vi "VAJ velocity in timing count.vi"(8 "dt":dbl, 9 "time":i32, 11 "Array":cluster{"Numeric":dbl, "Numeric":dbl}[](array[cluster])) -> (0 "t4?":bool, 2 "velocity(cm/s)":dbl, 4 "finish":bool)   [LabVIEW 2019]
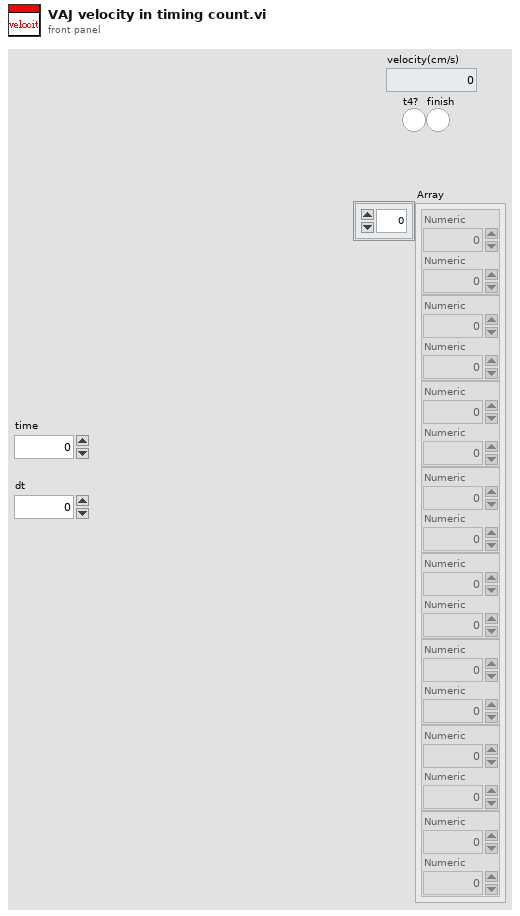
[diagram p1: front panel]
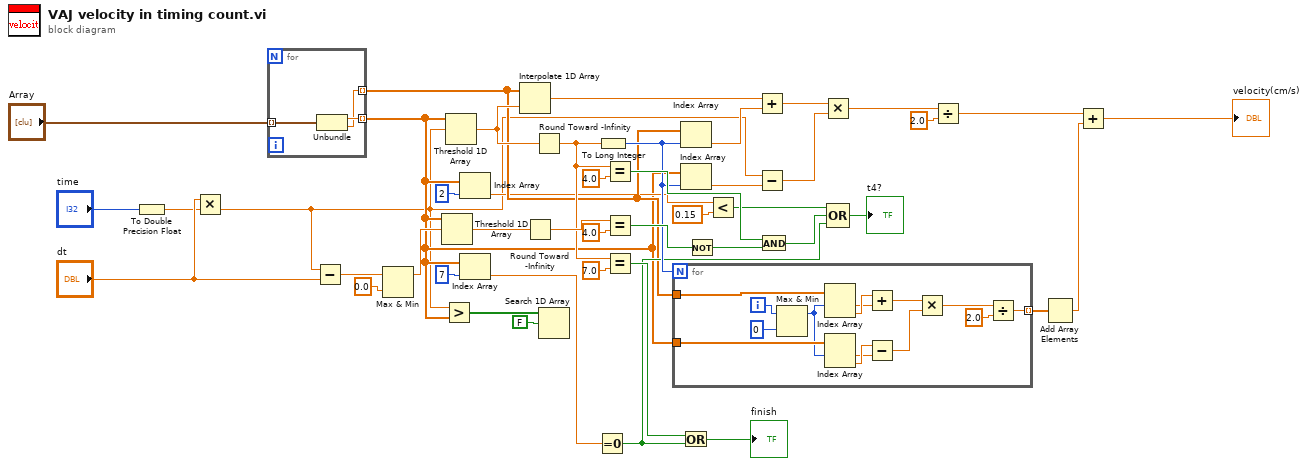
[diagram p0: block diagram]
diagram:
  n1 = To Double Precision Float(number="time") -> (double precision float=w1:dbl)
  n2 = Multiply(x="dt", y=w1) -> (x*y=w3:dbl)
  n3 = for {
    tunnel: "Array" -> [w48] mode=indexing
    tunnel: [w47] -> w4 mode=indexing
    tunnel: [w46] -> w9 mode=indexing
    n4 = Unbundle(w48) -> ("Numeric"=w47:dbl, "Numeric"=w46:dbl)
  }
  n5 = Subtract(x=w3, y="dt") -> (x-y=w35:dbl)
  n6 = Max & Min(x=w35, y=0.0) -> (max(x,y)=w24:dbl)  [unwired: 1 out]
  n7 = Threshold 1D Array(2:w24, 3:w4) -> (0:w34:dbl)  [unwired: 1 in]
  n8 = Greater?(x=w3, y=w4) -> (0:w44:bool[])
  n9 = Threshold 1D Array(2:w3, 3:w4) -> (0:w22:dbl)  [unwired: 1 in]
  n10 = Index Array(array=w4, index=2) -> (element=w7:dbl)
  n11 = Index Array(array=w4, index=7) -> (element=w11:dbl)
  n12 = Interpolate 1D Array(1:w22, 2:w9) -> (0:w18:dbl)
  n13 = Round Toward -Infinity(1:w34) -> (0:w27:dbl)
  n14 = Round Toward -Infinity(1:w22) -> (0:w20:dbl)
  n15 = Search 1D Array(1D array=w44, element=FALSE) -> ()  [unwired: 1 in, 1 out]
  n16 = Equal To 0?(x=w11) -> (x = 0?=w10:bool)
  n17 = To Long Integer(number=w20) -> (32bit integer=w19:i32)
  n18 = Equal?(x=w20, y=4.0) -> (x = y?=w30:bool)
  n19 = Equal?(x=w27, y=4.0) -> (x = y?=w31:bool)
  n20 = Equal?(x=w20, y=7.0) -> (x = y?=w25:bool)
  n21 = for {
    N: w19 -> [_]
    tunnel: w9 -> [w62]
    tunnel: w4 -> [w59]
    tunnel: [w52] -> w42 mode=indexing
    i -> [w49]
    n22 = Max & Min(x=w49, y=0) -> (max(x,y)=w50:i32)  [unwired: 1 out]
    n23 = Index Array(array=w62, index #1=w50) -> (element #1=w60:dbl, element #2=w61:dbl)  [unwired: 1 in]
    n24 = Index Array(array=w59, index #1=w50) -> (element #1=w57:dbl, element #2=w58:dbl)  [unwired: 1 in]
    n25 = Add(x=w61, y=w60) -> (x+y=w56:dbl)
    n26 = Subtract(x=w58, y=w57) -> (x-y=w55:dbl)
    n27 = Multiply(x=w56, y=w55) -> (x*y=w54:dbl)
    n28 = Divide(x=w54, y=2.0) -> (x/y=w52:dbl)
  }
  n29 = Index Array(array=w9, index=w19) -> (element=w17:dbl)
  n30 = Index Array(array=w4, index=w19) -> (element=w40:dbl)
  n31 = Or(x=w25, y=w10) -> (x .or. y?=→"finish":bool)
  n32 = Not(x=w31) -> (.not. x?=w29:bool)
  n33 = Less?(x=w7, y=0.15) -> (x < y?=w5:bool)
  n34 = Add(x=w18, y=w17) -> (x+y=w16:dbl)
  n35 = Subtract(x=w3, y=w40) -> (x-y=w39:dbl)
  n36 = And(x=w30, y=w29) -> (x .and. y?=w28:bool)
  n37 = Multiply(x=w16, y=w39) -> (x*y=w38:dbl)
  n38 = Compound Arithmetic op=OR(w5, w28, w10) -> (→"t4?":bool)
  n39 = Divide(x=w38, y=2.0) -> (x/y=w36:dbl)
  n40 = Add Array Elements(numeric array=w42) -> (sum=w41:dbl)
  n41 = Add(x=w36, y=w41) -> (x+y=→"velocity(cm/s)":dbl)
